vi "PathPlanner_Path_CreatePath_Worker1.vi"(6 "LargestWaypointIndex":dbl, 8 "GlobalConstraints":T5, 9 "ConstraintZones":T7[](array[typedef]), 10 "Waypoints":T6[](array[typedef]) {"nextControl"."Y" format="%14.3f"; "nextControl"."X" format="%14.3f"; "anchor"."Y" format="%14.3f"; "anchor"."X" format="%14.3f"; "prevControl"."Y" format="%14.3f"; "prevControl"."X" format="%14.3f"}, 11 "RotationTargets":T1[](array[typedef]) {"rotation"."SIN" format="%13.4f"; "rotation"."COS" format="%13.4f"; "rotation"."VALUE" format="%13.4f"}) -> (1 "pos":dbl, 2 "UnaddedTargets":T1[](array[typedef]) {"rotation"."SIN" format="%13.4f"; "rotation"."COS" format="%13.4f"; "rotation"."VALUE" format="%13.4f"}, 3 "Points":T3[](array[typedef]) {"RotationTarget"."rotation"."SIN" format="%13.4f"; "RotationTarget"."rotation"."COS" format="%13.4f"; "RotationTarget"."rotation"."VALUE" format="%13.4f"; "Position"."Y" format="%14.3f"; "Position"."X" format="%14.3f"})   [LabVIEW 2019, in "PathPlanner24.lvlib"]
uses:
  PathPlanner24.lvlib
  <vilib>/Rock Robotics/WPI/ThirdParty/JAS_Junk/TrajLib/Trajectory_Library.lvlib
  <vilib>/Rock Robotics/WPI/ThirdParty/JAS_Junk/TrajLib/TypeDef/ROTATION2D.ctl
  TypeDef/PathPlannerRotationTarget.ctl
  TypeDef/PathPlannerPathConstraints.ctl
  <vilib>/Rock Robotics/WPI/ThirdParty/JAS_Junk/TrajLib/TypeDef/TRANSLATION2D.ctl
  TypeDef/PathPlannerPathPoint.ctl
  TypeDef/PathPlannerConstraintsZone.ctl
  TypeDef/PathPlannerWaypoint.ctl
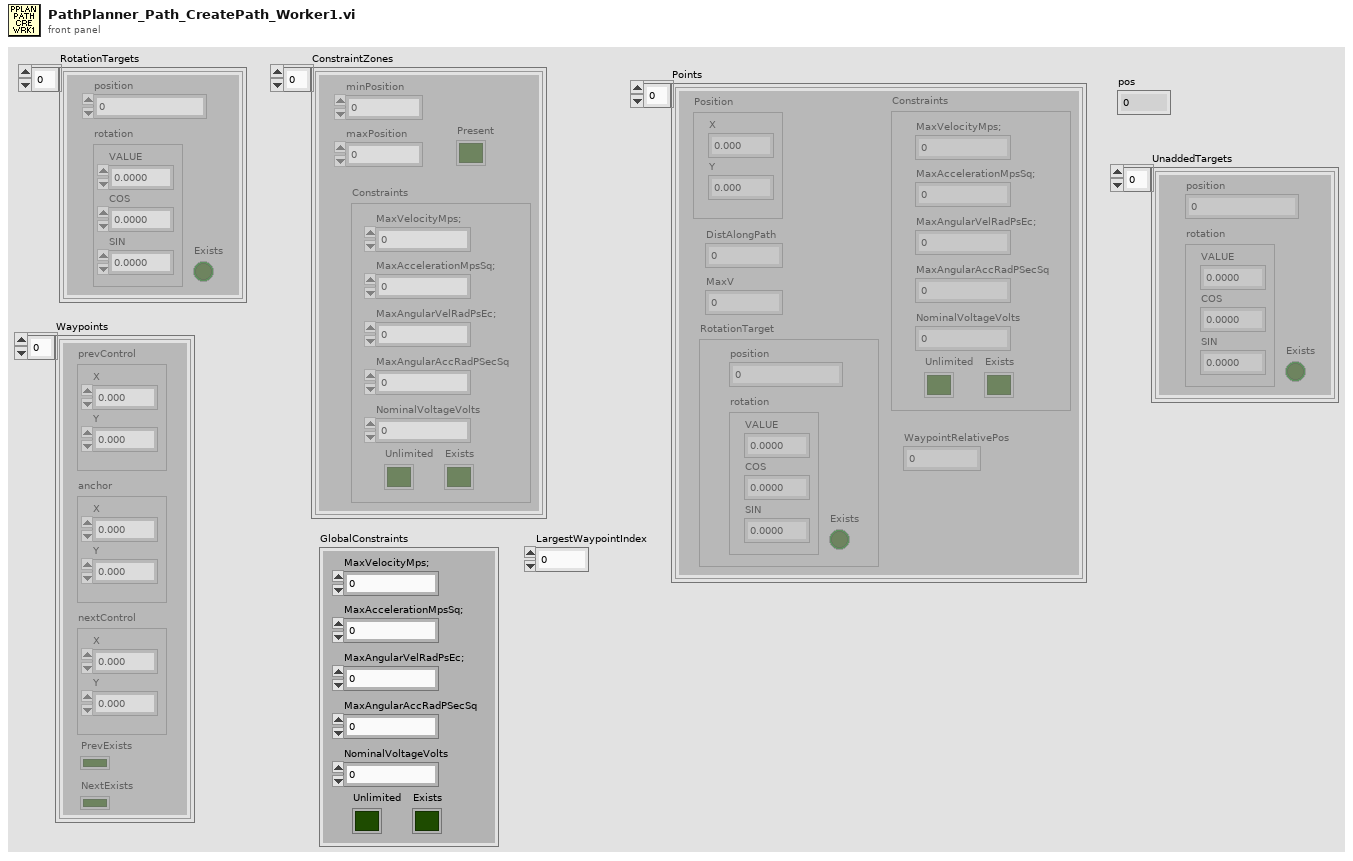
[diagram p1: front panel]
types:
  T1 = typedef "PathPlanner24.lvlib/PathPlannerRotationTarget.ctl" = cluster{"rotation":T2, "position":dbl, "Exists":bool}
  T2 = typedef "Trajectory_Library.lvlib/ROTATION2D.ctl" = cluster{"VALUE":dbl, "COS":dbl, "SIN":dbl}
  T3 = typedef "PathPlanner24.lvlib/PathPlannerPathPoint.ctl" = cluster{"Position":T4, "DistAlongPath":dbl, "MaxV":dbl, "Constraints":T5, "RotationTarget":T1, "WaypointRelativePos":dbl}
  T4 = typedef "Trajectory_Library.lvlib/TRANSLATION2D.ctl" = cluster{"X":dbl, "Y":dbl}
  T5 = typedef "PathPlanner24.lvlib/PathPlannerPathConstraints.ctl" = cluster{"MaxVelocityMps;":dbl, "MaxAccelerationMpsSq;":dbl, "MaxAngularVelRadPsEc;":dbl, "MaxAngularAccRadPSecSq":dbl, "Exists":bool, "Unlimited":bool, "NominalVoltageVolts":dbl}
  T6 = typedef "PathPlanner24.lvlib/PathPlannerWaypoint.ctl" = cluster{"prevControl":T4, "anchor":T4, "nextControl":T4, "PrevExists":bool, "NextExists":bool}
  T7 = typedef "PathPlanner24.lvlib/PathPlannerConstraintsZone.ctl" = cluster{"minPosition":dbl, "maxPosition":dbl, "Constraints":T5, "Present":bool}
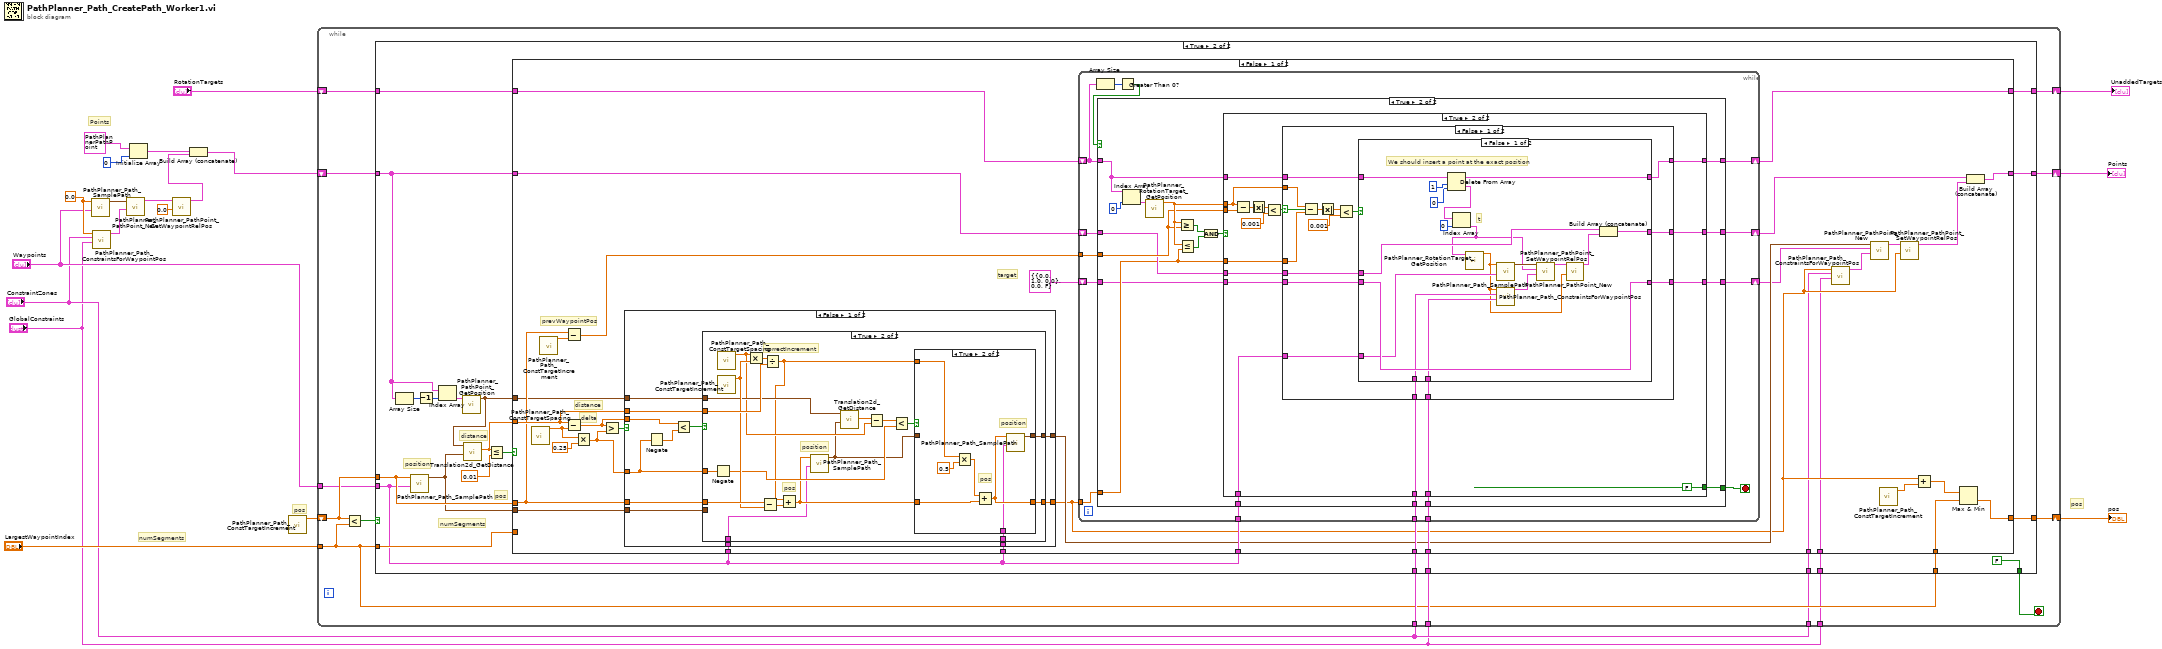
[diagram p0: block diagram]
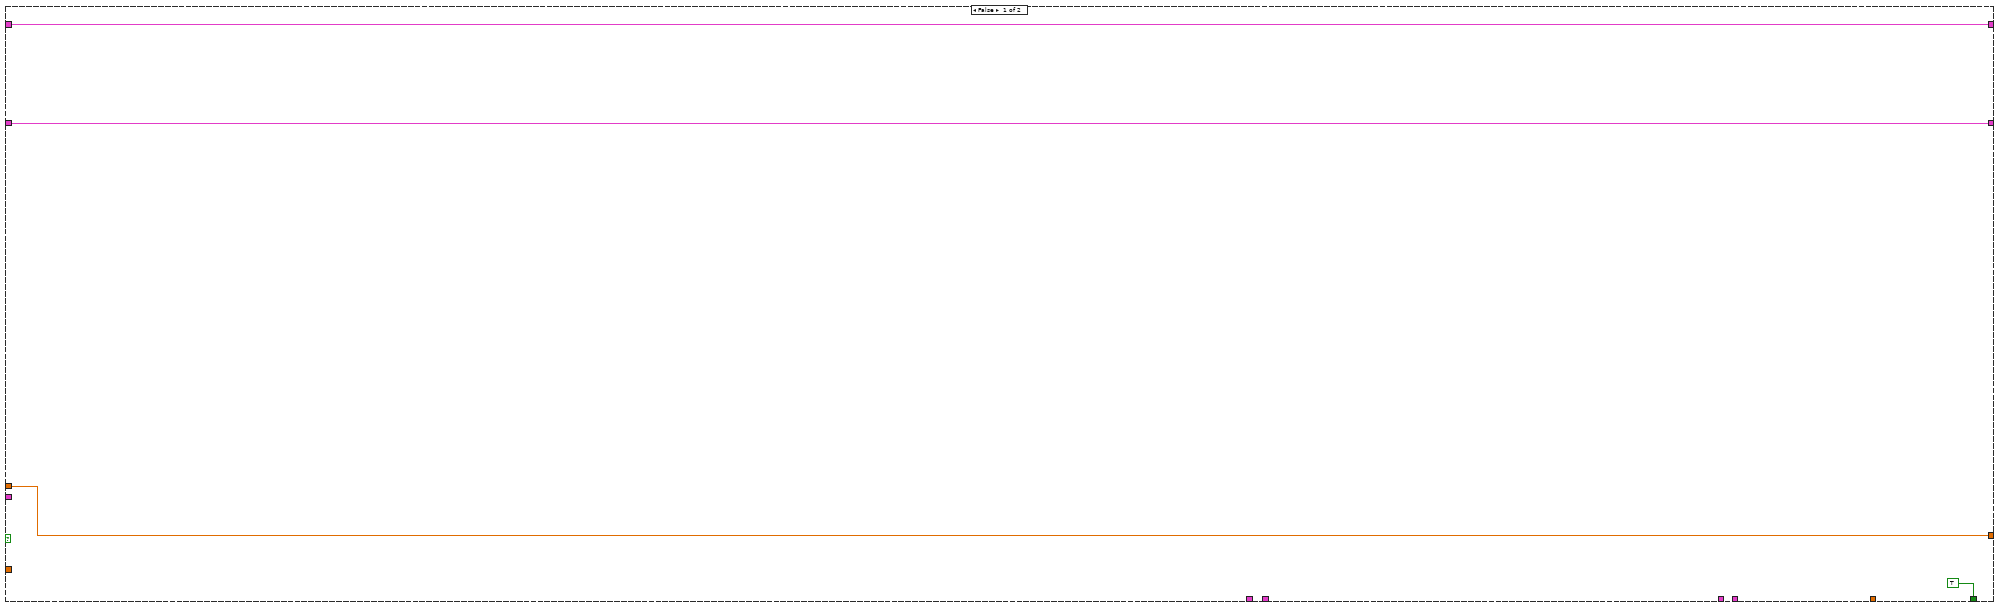
[diagram p2: hidden frame]
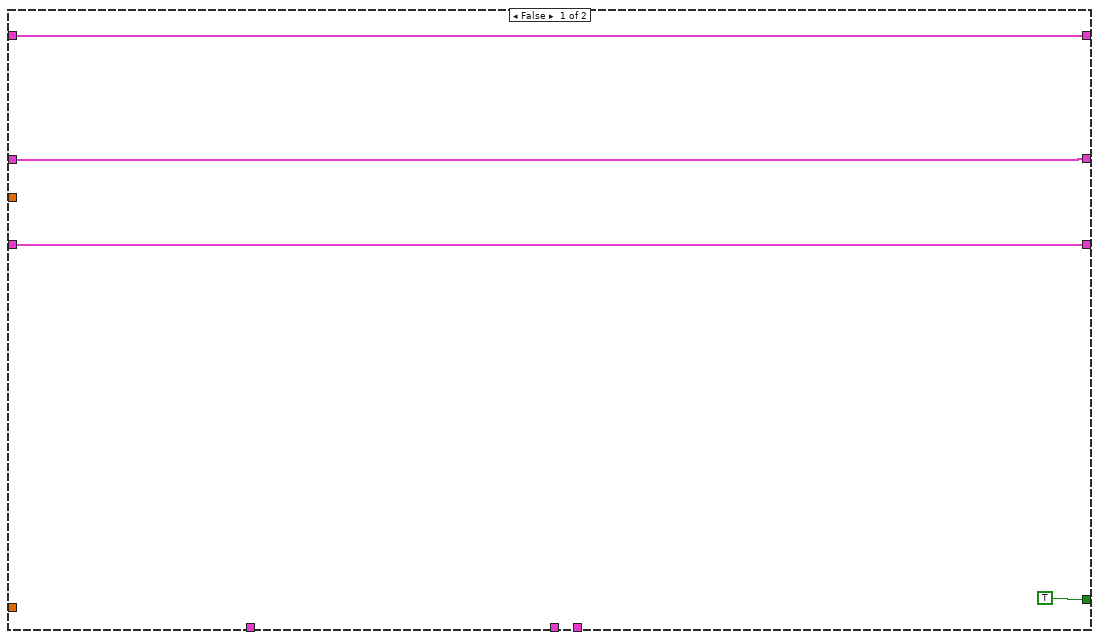
[diagram p3: hidden frame]
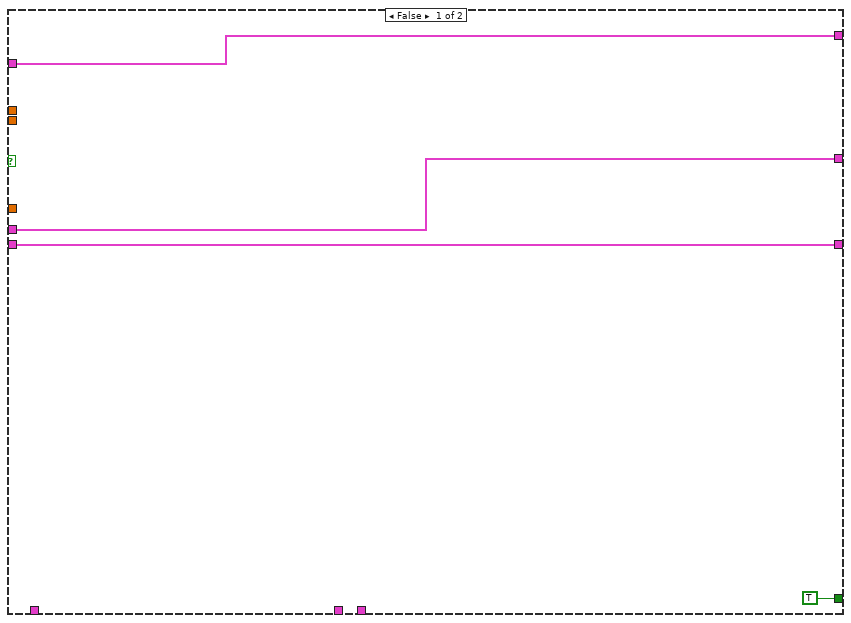
[diagram p4: hidden frame]
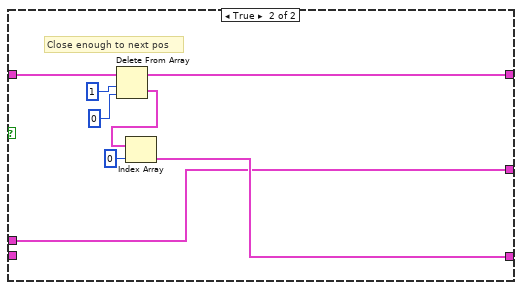
[diagram p5: hidden frame]
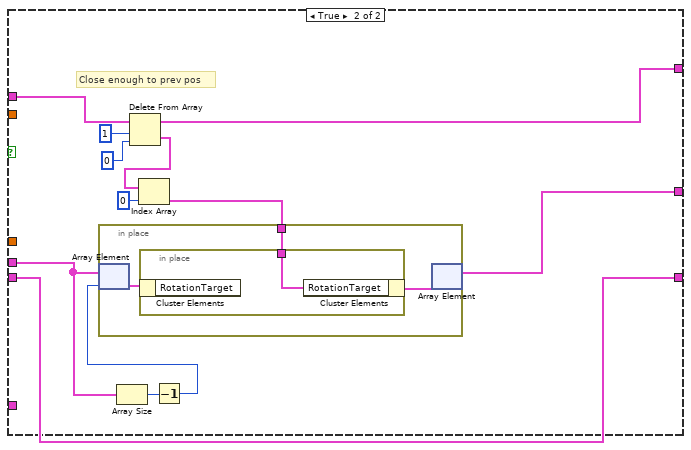
[diagram p6: hidden frame]
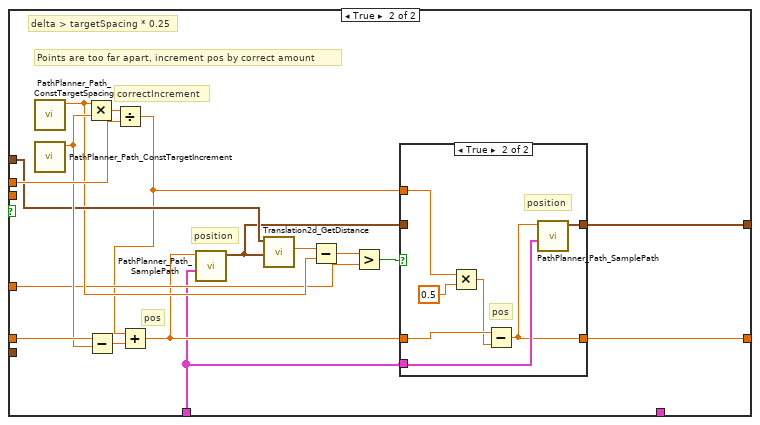
[diagram p9: hidden frame]
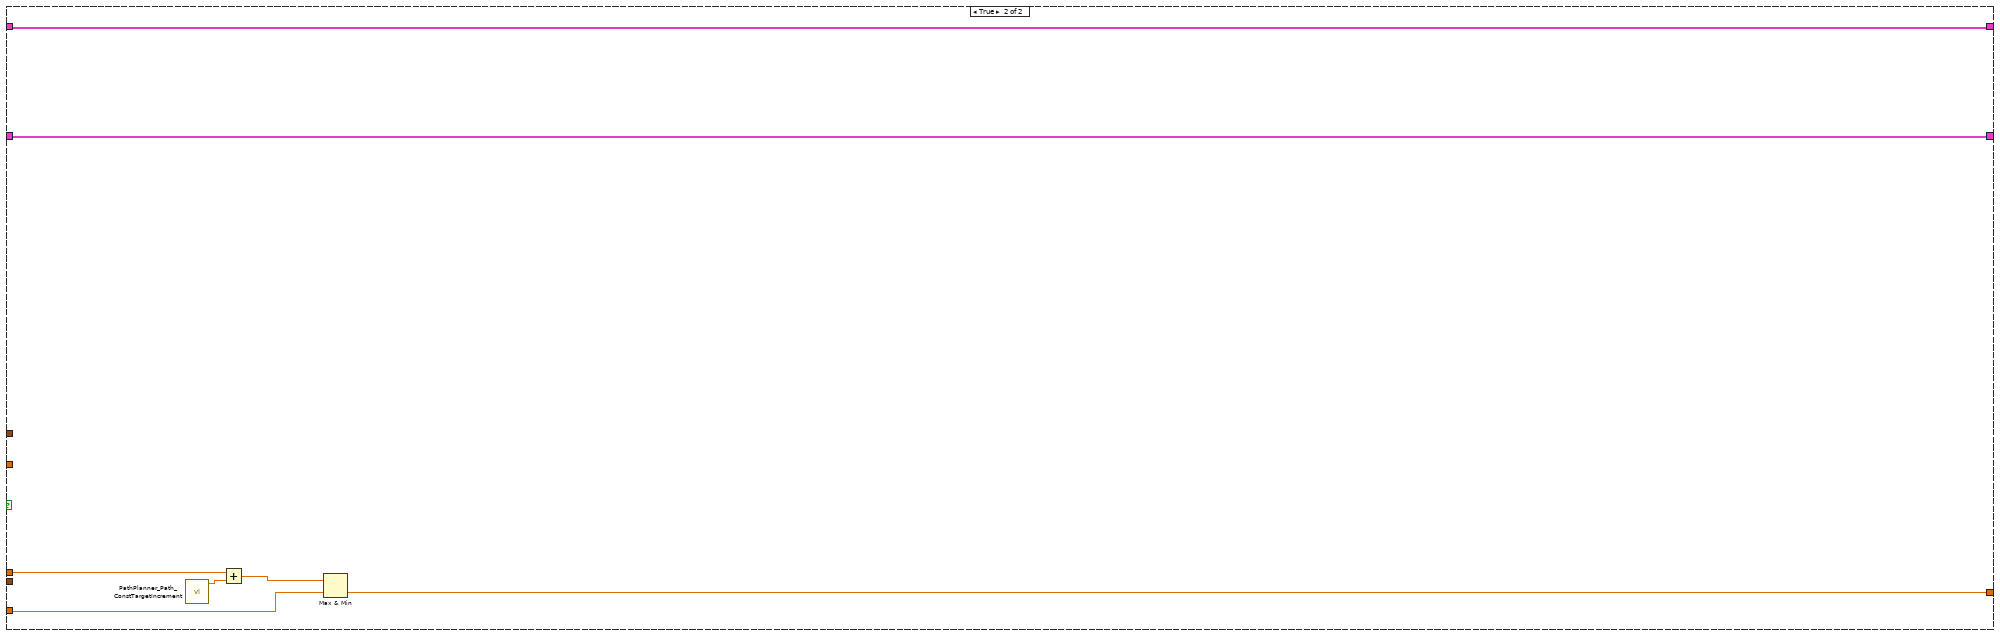
[diagram p11: hidden frame]
diagram:
  w11 = 0.0 ("WaypointRelativePos")
  # "numSegments"
  # "Points"
  # "pos"
  # "pos"
  n1 = call "PathPlanner_Path_SamplePath.vi"("Waypoints"="Waypoints", "WaypointRelativePos"=w11) -> ("Sample"=w12:T4)  [unwired: 9 in]
  n2 = call "PathPlanner_Path_ConstraintsForWaypointPos.vi"("GlobalConstraints"="GlobalConstraints", "ConstraintsZones"="ConstraintZones", "Pos"=w11) -> ("outPathPlannerPathConstraints"=w10:T5)  [unwired: 8 in]
  n3 = call "PathPlanner_PathPoint_New.vi"("Constraints"=w10, "Position"=w12) -> ("PathPlannerPoint"=w9:T3)  [unwired: 9 in]
  n4 = Initialize Array(T3 {"Position"={"X"=0.0, "Y"=0.0}, "DistAlongPath"=0.0, "MaxV"=9e+300, "Constraints"={"MaxVelocityMps;"=0.0, "MaxAccelerationMpsSq;"=0.0, "MaxAngularVelRadPsEc;"=0.0, "MaxAngularAccRadPSecSq"=0.0, "Exists"=FALSE, "Unlimited"=FALSE, "NominalVoltageVolts"=12.0}, "RotationTarget"={"rotation"={"VALUE"=0.0, "COS"=0.0, "SIN"=0.0}, "position"=1.0, "Exists"=FALSE}, "WaypointRelativePos"=0.0} ("PathPlannerPoint"), 0 ("dimension size")) -> (w13:T3[])
  n5 = call "PathPlanner_PathPoint_SetWaypointRelPos.vi"("WaypointRelativePos"=0.0, "PathPlannerPoint"=w9) -> ("outPathPlannerPoint"=w7:T3)  [unwired: 9 in]
  n6 = Build Array (concatenate)(w13, w7) -> (w6:T3[])
  n7 = call "PathPlanner_Path_ConstTargetIncrement.vi"() -> ("TargetIncrement"=w17:dbl)  [unwired: 11 in]
  n8 = while {
    shift-right: [w28] -> w16
    shift-left: w6 -> [w29]
    shift-right: [w26] -> w1
    shift-left: "RotationTargets" -> [w25]
    shift-right: [w27] -> w2
    shift-left: w17 -> [w31]
    tunnel: "LargestWaypointIndex" -> [w22]
    tunnel: "Waypoints" -> [w30]
    tunnel: "ConstraintZones" -> [w24]
    tunnel: "GlobalConstraints" -> [w23]
    tunnel: "ConstraintZones" -> [w21]
    tunnel: "GlobalConstraints" -> [w20]
    stop <- w32 stop-if-true
    n9 = Less?(x=w31, y=w22) -> (x < y?=w33:bool)
    n10 = case shown="True" w33 {
      tunnel: [TRUE FALSE] -> w32
      tunnel: w31 -> [w35 w52]
      tunnel: w30 -> [_ w44]
      tunnel: w29 -> [w36 w51]
      tunnel: [w36 w41] -> w28
      tunnel: [w35 w54] -> w27
      tunnel: w22 -> [_ w53]
      tunnel: [w34 w47] -> w26
      tunnel: w25 -> [w34 w46]
      tunnel: w24 -> [_ w43]
      tunnel: w23 -> [_ w42]
      tunnel: w22 -> [_ w40]
      tunnel: w21 -> [_ w39]
      tunnel: w20 -> [_ w38]
      frame False {
      }
      frame True {
        # "numSegments"
        # "pos"
        # "distance"
        # "position"
        n11 = Array Size(array=w51) -> (size(s)=w58:i32)
        n12 = call "PathPlanner_Path_SamplePath.vi"("Waypoints"=w44, "WaypointRelativePos"=w52) -> ("Sample"=w48:T4)  [unwired: 9 in]
        n13 = Decrement(x=w58) -> (x-1=w57:i32)
        n14 = Index Array(array=w51, index=w57) -> (element=w45:T3)
        n15 = call "PathPlanner_PathPoint_GetPosition.vi"("PathPlannerPoint"=w45) -> ("Position"=w49:T4)  [unwired: 10 in]
        n16 = call <vilib>:"Translation2d_GetDistance.vi"("other Translation"=w48, "In Translation"=w49) -> ("Distance"=w50:dbl)  [unwired: 9 in]
        n17 = Less Or Equal?(x=w50, y=0.01) -> (x <= y?=w55:bool)
        n18 = case shown="False" w55 {
          tunnel: [w66 w282] -> w54
          tunnel: w53 -> [_ w281]
          tunnel: w52 -> [w88 w280]
          tunnel: [w69 w277] -> w41
          tunnel: w51 -> [w79 w277]
          tunnel: w50 -> [w89 _]
          tunnel: w49 -> [w87 _]
          tunnel: w48 -> [w84 _]
          tunnel: [w82 w276] -> w47
          tunnel: w46 -> [w83 w276]
          tunnel: w44 -> [w78 _]
          tunnel: w44 -> [w77 _]
          tunnel: w44 -> [w76 _]
          tunnel: w43 -> [w75 _]
          tunnel: w42 -> [w74 _]
          tunnel: w40 -> [w65 _]
          tunnel: w39 -> [w61 _]
          tunnel: w38 -> [w60 _]
          frame False {
            # "target"
            # "distance"
            # "delta"
            # "prevWaypointPos"
            n19 = call "PathPlanner_Path_ConstTargetSpacing.vi"() -> ("TargetSpacing"=w92:dbl)  [unwired: 11 in]
            n20 = call "PathPlanner_Path_ConstTargetIncrement.vi"() -> ("TargetIncrement"=w93:dbl)  [unwired: 11 in]
            n21 = Subtract(x=w88, y=w93) -> (x-y=w80:dbl)
            n22 = Subtract(x=w89, y=w92) -> (x-y=w85:dbl)
            n23 = Multiply(x=w92, y=0.25) -> (x*y=w86:dbl)
            n24 = Greater?(x=w85, y=w86) -> (0:w90:bool)
            n25 = case shown="False" w90 {
              tunnel: w89 -> [w216 w265]
              tunnel: w88 -> [w215 w264]
              tunnel: w87 -> [w214 w261]
              tunnel: w86 -> [w213 w257]
              tunnel: w85 -> [w219 _]
              tunnel: [w211 w252] -> w68
              tunnel: [w212 w251] -> w63
              tunnel: w84 -> [w210 _]
              tunnel: w78 -> [w209 w250]
              tunnel: w77 -> [w208 _]
              frame False {
                n26 = Negate(x=w213) -> (-x=w218:dbl)
                n27 = Less?(x=w219, y=w218) -> (x < y?=w217:bool)
                n28 = case shown="True" w217 {
                  tunnel: w216 -> [_ w239]
                  tunnel: w215 -> [w221 w237]
                  tunnel: w214 -> [_ w234]
                  tunnel: w213 -> [_ w231]
                  tunnel: [w221 w227] -> w212
                  tunnel: [w220 w225] -> w211
                  tunnel: w210 -> [w220 _]
                  tunnel: w209 -> [_ w223]
                  tunnel: w208 -> [_ w222]
                  frame False {
                  }
                  frame True {
                    # "position"
                    # "pos"
                    # "correctIncrement"
                    n29 = Negate(x=w231) -> (-x=w230:dbl)
                    n30 = call "PathPlanner_Path_ConstTargetSpacing.vi"() -> ("TargetSpacing"=w233:dbl)  [unwired: 11 in]
                    n31 = call "PathPlanner_Path_ConstTargetIncrement.vi"() -> ("TargetIncrement"=w236:dbl)  [unwired: 11 in]
                    n32 = Multiply(x=w233, y=w236) -> (x*y=w240:dbl)
                    n33 = Subtract(x=w237, y=w236) -> (x-y=w238:dbl)
                    n34 = Divide(x=w240, y=w239) -> (x/y=w226:dbl)
                    n35 = Add(x=w226, y=w238) -> (x+y=w228:dbl)
                    n36 = call "PathPlanner_Path_SamplePath.vi"("Waypoints"=w223, "WaypointRelativePos"=w228) -> ("Sample"=w224:T4)  [unwired: 9 in]
                    n37 = call <vilib>:"Translation2d_GetDistance.vi"("other Translation"=w224, "In Translation"=w234) -> ("Distance"=w235:dbl)  [unwired: 9 in]
                    n38 = Subtract(x=w235, y=w233) -> (x-y=w232:dbl)
                    n39 = Less?(x=w232, y=w230) -> (x < y?=w229:bool)
                    n40 = case shown="True" w229 {
                      tunnel: w228 -> [w242 w247]
                      tunnel: [w242 w245] -> w227
                      tunnel: w226 -> [_ w246]
                      tunnel: [w241 w244] -> w225
                      tunnel: w224 -> [w241 _]
                      tunnel: w222 -> [_ w243]
                      frame False {
                      }
                      frame True {
                        # "position"
                        # "pos"
                        n41 = Multiply(x=w246, y=0.5) -> (x*y=w249:dbl)
                        n42 = Add(x=w249, y=w247) -> (x+y=w245:dbl)
                        n43 = call "PathPlanner_Path_SamplePath.vi"("Waypoints"=w243, "WaypointRelativePos"=w245) -> ("Sample"=w244:T4)  [unwired: 9 in]
                      }
                    }
                  }
                }
              }
              frame True {
                # "Points are too far apart, increment pos by correct amount"
                # "delta > targetSpacing * 0.25"
                # "position"
                # "pos"
                # "correctIncrement"
                n44 = call "PathPlanner_Path_ConstTargetSpacing.vi"() -> ("TargetSpacing"=w259:dbl)  [unwired: 11 in]
                n45 = call "PathPlanner_Path_ConstTargetIncrement.vi"() -> ("TargetIncrement"=w263:dbl)  [unwired: 11 in]
                n46 = Multiply(x=w259, y=w263) -> (x*y=w266:dbl)
                n47 = Subtract(x=w264, y=w263) -> (x-y=w262:dbl)
                n48 = Divide(x=w266, y=w265) -> (x/y=w255:dbl)
                n49 = Add(x=w255, y=w262) -> (x+y=w254:dbl)
                n50 = call "PathPlanner_Path_SamplePath.vi"("Waypoints"=w250, "WaypointRelativePos"=w254) -> ("Sample"=w253:T4)  [unwired: 9 in]
                n51 = call <vilib>:"Translation2d_GetDistance.vi"("other Translation"=w253, "In Translation"=w261) -> ("Distance"=w260:dbl)  [unwired: 9 in]
                n52 = Subtract(x=w260, y=w259) -> (x-y=w258:dbl)
                n53 = Greater?(x=w258, y=w257) -> (0:w256:bool)
                n54 = case shown="True" w256 {
                  tunnel: w255 -> [_ w274]
                  tunnel: w254 -> [w267 w270]
                  tunnel: [w267 w272] -> w251
                  tunnel: w250 -> [_ w273]
                  tunnel: [w268 w271] -> w252
                  tunnel: w253 -> [w268 _]
                  frame False {
                    # "pos"
                    # "position"
                  }
                  frame True {
                    # "position"
                    # "pos"
                    n55 = Multiply(x=w274, y=0.5) -> (x*y=w269:dbl)
                    n56 = Subtract(x=w270, y=w269) -> (x-y=w272:dbl)
                    n57 = call "PathPlanner_Path_SamplePath.vi"("Waypoints"=w273, "WaypointRelativePos"=w272) -> ("Sample"=w271:T4)  [unwired: 9 in]
                  }
                }
              }
            }
            n58 = while {
              tunnel: w63 -> [w105]
              tunnel: w80 -> [w104]
              shift-right: [w107] -> w82
              shift-left: w83 -> [w102]
              shift-right: [w98] -> w70
              shift-left: w79 -> [w99]
              shift-right: [w97] -> w67
              shift-left: T1 {"rotation"={"VALUE"=0.0, "COS"=1.0, "SIN"=0.0}, "position"=0.0, "Exists"=FALSE} ("RotationTarget") -> [w106]
              tunnel: w76 -> [w96]
              tunnel: w75 -> [w95]
              tunnel: w74 -> [w94]
              stop <- w100 stop-if-true
              n59 = Array Size(array=w102) -> (size(s)=w103:i32)
              n60 = Greater Than 0?(x=w103) -> (x > 0?=w101:bool)
              n61 = case shown="True" w101 {
                tunnel: w102 -> [w110 w126]
                tunnel: [w110 w125] -> w107
                tunnel: w106 -> [w108 w116]
                tunnel: w105 -> [_ w117]
                tunnel: w104 -> [_ w120]
                tunnel: [TRUE w123] -> w100
                tunnel: w99 -> [w109 w119]
                tunnel: [w109 w118] -> w98
                tunnel: [w108 w115] -> w97
                tunnel: w96 -> [_ w114]
                tunnel: w95 -> [_ w113]
                tunnel: w94 -> [_ w112]
                frame False {
                }
                frame True {
                  n62 = Index Array(array=w126, index=0) -> (element=w128:T1)
                  n63 = call "PathPlanner_RotationTarget_GetPosition.vi"("RotationTarget"=w128) -> ("position"=w121:dbl)  [unwired: 9 in, 1 out]
                  n64 = Greater Or Equal?(x=w121, y=w120) -> (x >= y?=w122:bool)
                  n65 = Less Or Equal?(x=w121, y=w117) -> (x <= y?=w127:bool)
                  n66 = And(x=w122, y=w127) -> (x .and. y?=w124:bool)
                  n67 = case shown="True" w124 {
                    tunnel: w126 -> [w132 w144]
                    tunnel: [w132 w143] -> w125
                    tunnel: [TRUE FALSE] -> w123
                    tunnel: w121 -> [_ w140]
                    tunnel: w120 -> [_ w148]
                    tunnel: w119 -> [w131 w142]
                    tunnel: [w131 w141] -> w118
                    tunnel: w117 -> [_ w139]
                    tunnel: w116 -> [w130 w138]
                    tunnel: [w130 w137] -> w115
                    tunnel: w114 -> [_ w136]
                    tunnel: w113 -> [_ w135]
                    tunnel: w112 -> [_ w134]
                    frame False {
                    }
                    frame True {
                      n68 = Subtract(x=w140, y=w148) -> (x-y=w149:dbl)
                      n69 = Absolute Value(x=w149) -> (abs(x)=w147:dbl)
                      n70 = Less?(x=w147, y=0.001) -> (x < y?=w145:bool)
                      n71 = case shown="False" w145 {
                        tunnel: w144 -> [w159 w203]
                        tunnel: [w158 w200] -> w143
                        tunnel: w142 -> [w155 w196]
                        tunnel: [w156 w193] -> w141
                        tunnel: w140 -> [w162 _]
                        tunnel: w139 -> [w161 _]
                        tunnel: w138 -> [w154 w192]
                        tunnel: [w157 w192] -> w137
                        tunnel: w136 -> [w153 _]
                        tunnel: w135 -> [w152 _]
                        tunnel: w134 -> [w151 _]
                        frame False {
                          n72 = Subtract(x=w162, y=w161) -> (x-y=w165:dbl)
                          n73 = Absolute Value(x=w165) -> (abs(x)=w164:dbl)
                          n74 = Less?(x=w164, y=0.001) -> (x < y?=w160:bool)
                          n75 = case shown="False" w160 {
                            tunnel: w159 -> [w179 w187]
                            tunnel: [w178 w186] -> w158
                            tunnel: [w177 w185] -> w157
                            tunnel: [w175 w184] -> w156
                            tunnel: w155 -> [w176 w184]
                            tunnel: w154 -> [w177 _]
                            tunnel: w153 -> [w174 _]
                            tunnel: w152 -> [w171 _]
                            tunnel: w151 -> [w170 _]
                            frame False {
                              # "t"
                              # "We should insert a point at the exact position"
                              n76 = Delete From Array(array=w179, length=1, index=0) -> (deleted portion=w181:T1[], array with subset deleted=w178:T1[])
                              n77 = Index Array(array=w181, index=0) -> (element=w172:T1)
                              n78 = call "PathPlanner_RotationTarget_GetPosition.vi"("RotationTarget"=w172) -> ("position"=w167:dbl)  [unwired: 9 in, 1 out]
                              n79 = call "PathPlanner_Path_SamplePath.vi"("Waypoints"=w174, "WaypointRelativePos"=w167) -> ("Sample"=w173:T4)  [unwired: 9 in]
                              n80 = call "PathPlanner_Path_ConstraintsForWaypointPos.vi"("GlobalConstraints"=w170, "ConstraintsZones"=w171, "Pos"=w167) -> ("outPathPlannerPathConstraints"=w169:T5)  [unwired: 8 in]
                              n81 = call "PathPlanner_PathPoint_New.vi"("Constraints"=w169, "RotationTarget"=w172, "Position"=w173) -> ("PathPlannerPoint"=w168:T3)  [unwired: 8 in]
                              n82 = call "PathPlanner_PathPoint_SetWaypointRelPos.vi"("WaypointRelativePos"=w167, "PathPlannerPoint"=w168) -> ("outPathPlannerPoint"=w166:T3)  [unwired: 9 in]
                              n83 = Build Array (concatenate)(w176, w166) -> (w175:T3[])
                            }
                            frame True {
                              # "Close enough to next pos"
                              n84 = Delete From Array(array=w187, length=1, index=0) -> (deleted portion=w189:T1[], array with subset deleted=w186:T1[])
                              n85 = Index Array(array=w189, index=0) -> (element=w185:T1)
                            }
                          }
                        }
                        frame True {
                          # "Close enough to prev pos"
                          n86 = Array Size(array=w196) -> (size(s)=w197:i32)
                          n87 = Delete From Array(array=w203, length=1, index=0) -> (deleted portion=w199:T1[], array with subset deleted=w200:T1[])
                          n88 = Index Array(array=w199, index=0) -> (element=w194:T1)
                          n89 = Decrement(x=w197) -> (x-1=w195:i32)
                          n90 = in-place {
                            in-place-border: w194 -> [w204]
                            n91 = in-place-array #1(w196, w195) -> (w206:T3)
                            n92 = in-place {
                              in-place-border: w204 -> [w207]
                              n93 = in-place-cluster #2(w206) -> ()  [unwired: 1 out]
                              n94 = in-place-cluster #2("RotationTarget"=w207) -> (w205:T3)
                            }
                            n95 = in-place-array #1(w205) -> (w193:T3[])  [unwired: 1 out]
                          }
                        }
                      }
                    }
                  }
                }
              }
            }
            n96 = call "PathPlanner_Path_ConstraintsForWaypointPos.vi"("GlobalConstraints"=w60, "ConstraintsZones"=w61, "Pos"=w63) -> ("outPathPlannerPathConstraints"=w73:T5)  [unwired: 8 in]
            n97 = call "PathPlanner_PathPoint_New.vi"("Constraints"=w73, "RotationTarget"=w67, "Position"=w68) -> ("PathPlannerPoint"=w72:T3)  [unwired: 8 in]
            n98 = call "PathPlanner_Path_ConstTargetIncrement.vi"() -> ("TargetIncrement"=w62:dbl)  [unwired: 11 in]
            n99 = call "PathPlanner_PathPoint_SetWaypointRelPos.vi"("WaypointRelativePos"=w63, "PathPlannerPoint"=w72) -> ("outPathPlannerPoint"=w71:T3)  [unwired: 9 in]
            n100 = Add(x=w63, y=w62) -> (x+y=w64:dbl)
            n101 = Max & Min(x=w64, y=w65) -> (min(x,y)=w66:dbl)  [unwired: 1 out]
            n102 = Build Array (concatenate)(w70, w71) -> (w69:T3[])
          }
          frame True {
            n103 = call "PathPlanner_Path_ConstTargetIncrement.vi"() -> ("TargetIncrement"=w279:dbl)  [unwired: 11 in]
            n104 = Add(x=w280, y=w279) -> (x+y=w278:dbl)
            n105 = Max & Min(x=w278, y=w281) -> (min(x,y)=w282:dbl)  [unwired: 1 out]
          }
        }
      }
    }
  }
  "Points" <- w16
  "pos" <- w2
  "UnaddedTargets" <- w1
